vi "Actor Setup.vi"(10 "Actor":refnum<class "Actor.lvclass">, 11 "Dev Actor in":refnum<class "Dev Actor.lvclass">) -> (0 "error out":errorcluster, 3 "Dev Actor out":refnum<class "Dev Actor.lvclass">)   [LabVIEW 2021, in "Dev Actor.lvlib" / "Dev Actor.lvclass"]
uses:
  Dev Actor.lvclass
  src/LVCAM/LVCAM/Actor/Actor.lvclass
  Dev Actor Panel/Dev Actor Panel.lvclass
  C:/git/jettl/src/Panel/Panel.lvclass
  Dev Actor.lvclass/Dev Actor.ctl
  Panel/Panel.lvclass
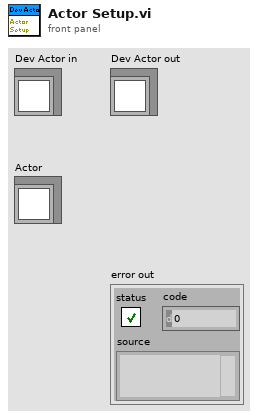
[diagram p1: front panel]
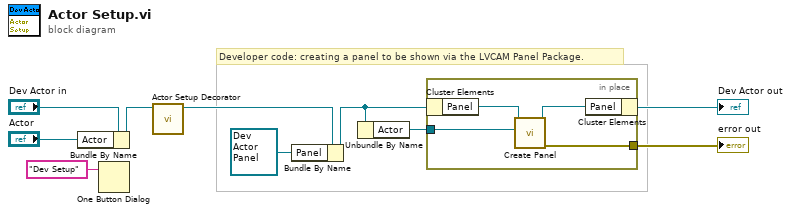
[diagram p0: block diagram]
diagram:
  # "Developer code: creating a panel to be shown via the LVCAM Panel Package."
  n1 = Bundle By Name(cluster="Dev Actor in", "Actor"="Actor") -> (w2:refnum<class "Dev Actor.lvclass">)
  n2 = One Button Dialog(message="Dev Setup") -> ()  [unwired: 1 in, 1 out]
  n3 = call "Actor Setup Decorator.vi"("Dev Actor in"=w2) -> ("Dev Actor out"=w1:refnum<class "Dev Actor.lvclass">)  [unwired: 9 in, 1 out]
  n4 = Bundle By Name(cluster=w1, "Panel"=refnum<class "Dev Actor Panel.lvclass"> refnum ("ABD Panel.lvclass")) -> (w4:refnum<class "Dev Actor.lvclass">)
  n5 = Unbundle By Name(w4) -> ("Actor"=w5:refnum<class "Actor.lvclass">)
  n6 = in-place {
    in-place-border: [w12] -> w6
    in-place-border: w5 -> [w11]
    n7 = in-place-cluster #1(w4) -> ("Panel"=w14:refnum<class "Panel.lvclass">)
    n8 = call "Create Panel.vi"("Actor"=w11, "Panel in"=w14) -> ("error out"=w12:errorcluster, "Panel out"=w13:refnum<class "Panel.lvclass">)  [unwired: 8 in]
    n9 = in-place-cluster #1("Panel"=w13) -> (→"Dev Actor out":refnum<class "Dev Actor.lvclass">)
  }
  "error out" <- w6
